vi "Channel list to pattern.vi"(10 "Outputs":i32=52, 11 "List":i32[](array[numeric])) -> (2 "Pattern":u32[](array[numeric]))   [LabVIEW 2020, in "Pickering.lvlib" / "PIPX40 Relay.lvclass"]
uses:
  PIPX40 Relay.lvclass
  PIPX40 Relay.lvclass/PIPX40 Relay.ctl
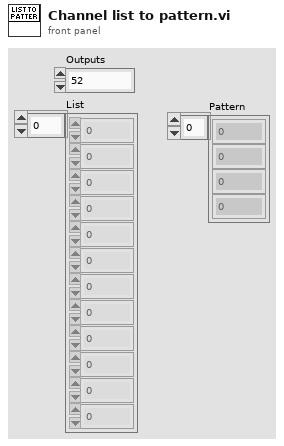
[diagram p1: front panel]
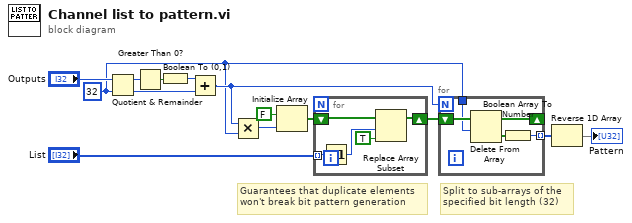
[diagram p0: block diagram]
diagram:
  w1 = 32 ("y")
  # "Split to sub-arrays of the\nspecified bit length (32)"
  # "Guarantees that duplicate elements\nwon't break bit pattern generation"
  n1 = Quotient & Remainder(x="Outputs", y=w1) -> (x-y*floor(x/y)=w6:i32, floor(x/y)=w3:i32)
  n2 = Greater Than 0?(x=w6) -> (x > 0?=w5:bool)
  n3 = Boolean To (0,1)(Boolean=w5) -> (0, 1=w4:i16)
  n4 = Add(x=w4, y=w3) -> (x+y=w2:i32)
  n5 = Multiply(x=w2, y=w1) -> (x*y=w9:i32)
  n6 = Initialize Array(FALSE, w9) -> (w13:bool[])
  n7 = for {
    tunnel: "List" -> [w17] mode=indexing
    shift-right: [w18] -> w11
    shift-left: w13 -> [w19]
    n8 = Decrement(x=w17) -> (x-1=w16:i32)
    n9 = Replace Array Subset(array=w19, new element=TRUE, index=w16) -> (w18:bool[])
  }
  n10 = for {
    N: w2 -> [_]
    tunnel: [w22] -> w10 mode=indexing
    shift-right: [w21] -> _
    shift-left: w11 -> [w24]
    tunnel: w1 -> [w20]
    n11 = Delete From Array(array=w24, length=w20) -> (deleted portion=w23:bool[], array with subset deleted=w21:bool[])  [unwired: 1 in]
    n12 = Boolean Array To Number(Boolean array=w23) -> (number=w22:u32)
  }
  n13 = Reverse 1D Array(array=w10) -> (reversed array=→"Pattern":u32[])
